vi "UnMarshall.vi"(7 "Type":variant, 8 "error in (no error)":errorcluster, 10 "String":string, 11 "Serializer in":refnum<class "Serializer.PlainText.lvclass">) -> (0 "error out":errorcluster, 2 "Variant":variant, 3 "Serializer out":refnum<class "Serializer.PlainText.lvclass">)   [LabVIEW 2013, in "CfgManager.Text.lvlib" / "Serializer.PlainText.lvclass"]
uses:
  Serializer.PlainText.lvclass
  <vilib>/LabVIEW Open Source/Data Manipulation/TypeDescriptor/TypeDescriptor_GetName.vi
  <vilib>/LabVIEW Open Source/Data Manipulation/TypeDescriptor/TypeDescriptor_GetPString.vi
  <vilib>/LabVIEW Open Source/Data Manipulation/Variant/OpenVariant.lvlib
  <vilib>/Utility/VariantDataType/VariantType.lvlib
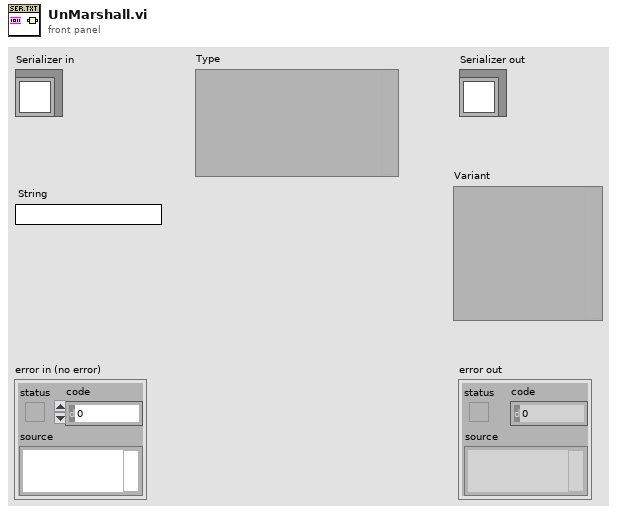
[diagram p1: front panel]
types:
  T1 = typedef "VariantType.lvlib/Type.ctl" = enum8{"Invalid Type", "Void", "I8", "I16", "I32", "I64", "U8", "U16", "U32", "U64", "Single Float", "Double Float", "Extended Float", "Single Complex", "Double Complex", "Extended Complex", "Enum U8", "Enum U16", "Enum U32", "Enum U64", "Single Float With Unit", "Double Float With Unit", "Extended Float With Unit", "Single Complex with Unit", "Double Complex with Unit", "Extended Complex with Unit", "Boolean", "String", "Path", "Picture", "Tag", "Array", "Cluster", "Variant", "LV Variant", "Waveform", "Timestamp", "Digital Waveform", "Digital Data", "ExpressData", "Refnum", "External Data", "VI", "Poly VI", "LabVIEW Class Instance", "Fixed Point"}
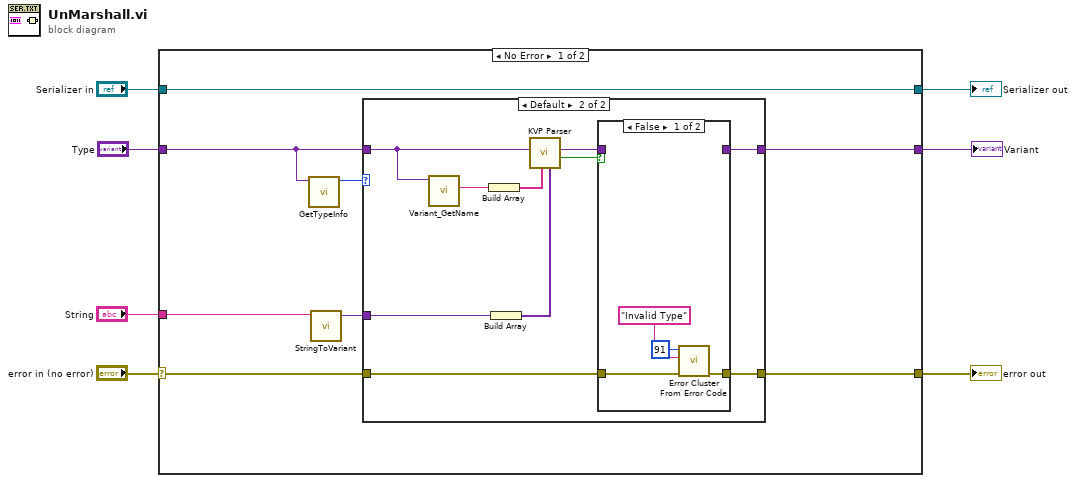
[diagram p0: block diagram]
diagram:
  n1 = case shown="No Error" "error in (no error)" {
    selector: "error in (no error)" -> [w9 w35]
    tunnel: [w8 w35] -> w6
    tunnel: [w15 w34] -> w4
    tunnel: "Serializer in" -> [w15 w34]
    tunnel: [w12 _] -> w3
    tunnel: "Type" -> [w11 _]
    tunnel: "String" -> [w14 _]
    frame No Error {
      n2 = call <vilib>:"GetTypeInfo.vi"("Variant"=w11) -> ("Type Enum"=w10:T1)  [unwired: 6 in, 4 out]
      n3 = call "StringToVariant.vi"("String-formatted Value"=w14) -> ("Variant-formatted Value"=w13:variant)  [unwired: 9 in, 1 out]
      n4 = case shown="Default" w10 {
        tunnel: w13 -> [w17 w25]
        tunnel: [w17 w20] -> w12
        tunnel: w11 -> [_ w23]
        tunnel: w9 -> [w16 w18]
        tunnel: [w16 w19] -> w8
        frame "Void" {
        }
        frame Default {
          n5 = call <vilib>:"Variant_GetName.vi"("Variant"=w23) -> ("Name"=w27:string)  [unwired: 8 in, 2 out]
          n6 = Build Array(w27) -> (w26:string[])
          n7 = Build Array(w25) -> (w24:variant[])
          n8 = call <vilib>:"KVP Parser.vi"("Values"=w24, "Keys"=w26, "Default Value"=w23) -> ("any found?"=w22:bool, "Value"=w21:variant)  [unwired: 5 in, 2 out]
          n9 = case shown="False" w22 {
            tunnel: w21 -> [_ w33]
            tunnel: [_ w33] -> w20
            tunnel: [w31 w32] -> w19
            tunnel: w18 -> [w30 w32]
            frame False {
              n10 = call <vilib>:"Error Cluster From Error Code.vi"("error in (no error)"=w30, "error message (\"\")"="Invalid Type", "error code (0)"=91) -> ("error out"=w31:errorcluster)  [unwired: 6 in]
            }
            frame True {
            }
          }
        }
      }
    }
    frame Error {
    }
  }
  "error out" <- w6
  "Serializer out" <- w4
  "Variant" <- w3
